vi "DSF.Engine.Memory.ObjectPool.Set Index FIFO.vi"(8 "error in (no error)":errorcluster, 10 "Index FIFO":refnum<k33>, 11 "ObjectPool in":refnum<class "DSF.Engine.Memory.ObjectPool.lvclass">) -> (0 "error out":errorcluster, 3 "ObjectPool out":refnum<class "DSF.Engine.Memory.ObjectPool.lvclass">)   [LabVIEW 2016, in "DSF.Engine.lvlib" / "DSF.Engine.Memory.ObjectPool.lvclass"]
uses:
  DSF.Engine.Memory.ObjectPool.lvclass
  DSF.Engine.Memory.ObjectPool.lvclass/DSF.Engine.Memory.ObjectPool.ctl
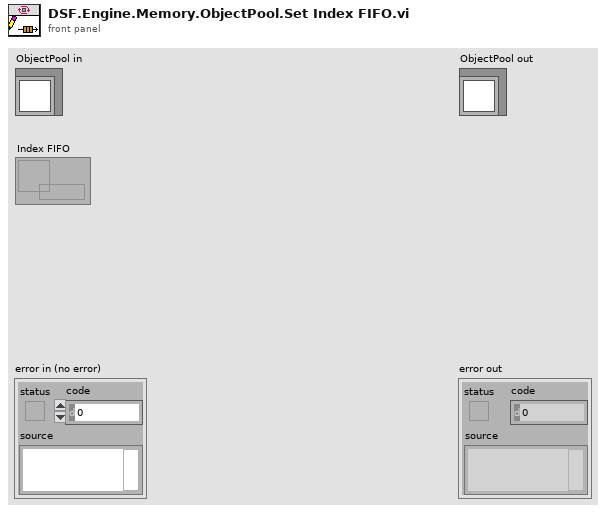
[diagram p1: front panel]
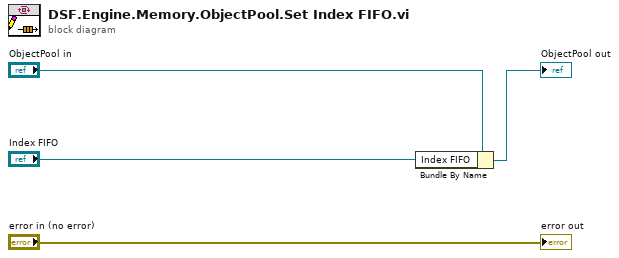
[diagram p0: block diagram]
diagram:
  n1 = Bundle By Name(cluster="ObjectPool in", "Index FIFO"="Index FIFO") -> (→"ObjectPool out":refnum<class "DSF.Engine.Memory.ObjectPool.lvclass">)
  "error out" <- "error in (no error)"
